vi "Set Element Read Position.vi"(6 "Allow Pass Head":bool, 8 "error in (no error)":errorcluster, 9 "Element Index Offset":i32, 10 "Read Position (Newest)":T1=enum."Newest", 11 "CIPC Reference":u64) -> (0 "error out":errorcluster)   [LabVIEW 2021, in "CIF_NI_CIPC.lvlib"]
uses:
  CIF_NI_CIPC.lvlib
  TypeDefs/Read Position.ctl
  <vilib>/Utility/error.llb/Trim Whitespace.vi
  <vilib>/Utility/error.llb/Error Cluster From Error Code.vi
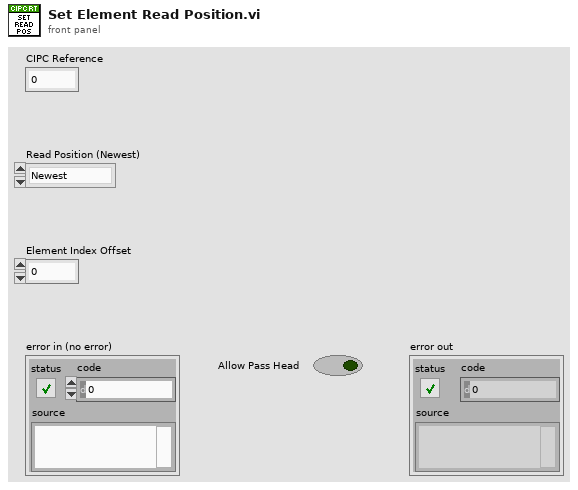
[diagram p1: front panel]
types:
  T1 = typedef "CIF_NI_CIPC.lvlib/Read Position.ctl" = enum16{"Next", "Newest", "Oldest", "Next Available", "Absolute"}
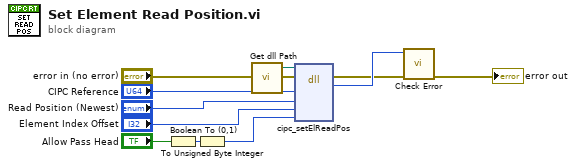
[diagram p0: block diagram]
diagram:
  n1 = Boolean To (0,1)(Boolean="Allow Pass Head") -> (0, 1=w4:i16)
  n2 = To Unsigned Byte Integer(number=w4) -> (unsigned 8bit integer=w2:u8)
  n3 = call "Get dll Path.vi"() -> ("appended path"=w1:path)  [unwired: 5 in]
  n4 = dll-call lib="libnicipc.*" fn="cipc_setElReadPos"(path in=w1, error in="error in (no error)", "cipc_buffer_ref"="CIPC Reference", "read_pos"="Read Position (Newest)", "el_index_offs"="Element Index Offset", "allowPassHead"=w2) -> (error out=w9:errorcluster, "return type"=w10:i32)  [unwired: 5 in, 1 out]
  n5 = call "Check Error.vi"("error in (no error)"=w9, "Error Code"=w10) -> ("error out"=→"error out":errorcluster)  [unwired: 9 in]
